vi "Latest File Check.vi"(5 "Target File Path":string, 7 "Initial File Path":string, 8 "error in (no error)":errorcluster, 9 "Matched Folder":string, 10 "Initial body in":string, 11 "Refnum in":T1) -> (0 "error out":errorcluster, 1 "body out":string, 2 "File Path Out":string, 3 "Refnum out":T1)   [LabVIEW 2019]
uses:
  <vilib>/httpClient/ClientHandle.ctl
  <vilib>/httpClient/LabVIEWHTTPClient.lvlib
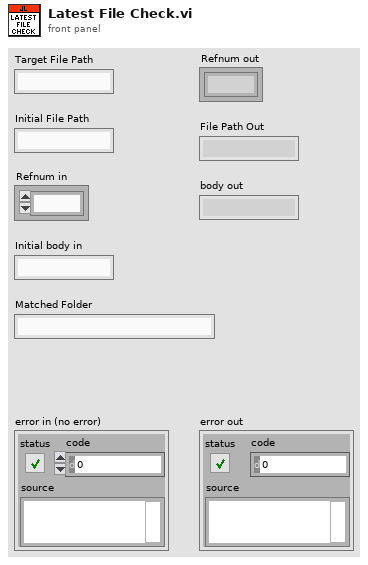
[diagram p1: front panel]
types:
  T1 = typedef "LabVIEWHTTPClient.lvlib/ClientHandle.ctl" = refnum<k1>
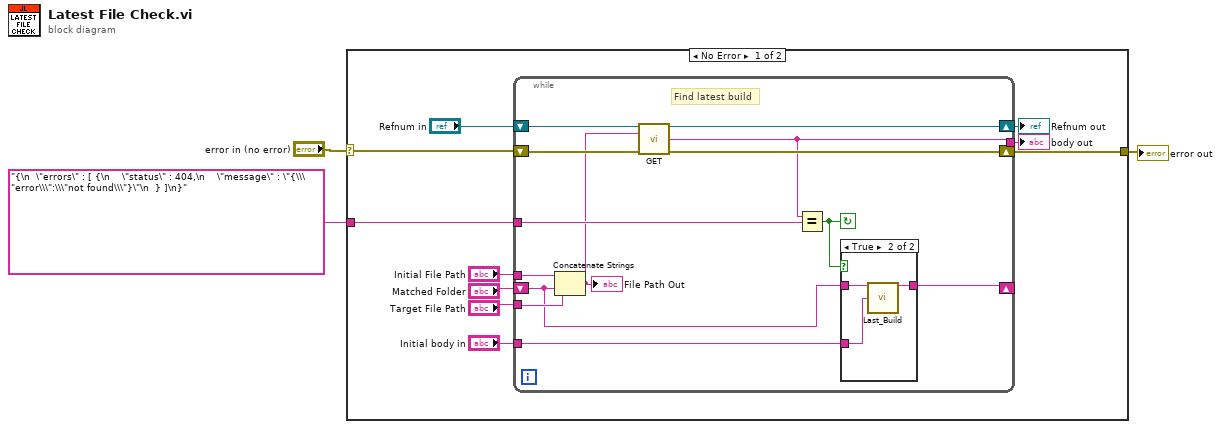
[diagram p0: block diagram]
diagram:
  n1 = case shown="No Error" "error in (no error)" {
    selector: "error in (no error)" -> [w6 w31]
    tunnel: "{\n  \"errors\" : [ {\n    \"status\" : 404,\n    \"message\" : \"{\\\"error\\\":\\\"not found\\\"}\"\n  } ]\n}" -> [w7 _]
    tunnel: [w4 w31] -> w1
    frame No Error {
      n2 = while {
        tunnel: "Initial File Path" -> [w26]
        shift-right: [w24] -> w4
        shift-left: w6 -> [w25]
        shift-right: [w21] -> w11
        shift-left: "Refnum in" -> [w22]
        tunnel: "Target File Path" -> [w23]
        shift-right: [w19] -> _
        shift-left: "Matched Folder" -> [w14]
        tunnel: "Initial body in" -> [w18]
        tunnel: w7 -> [w17]
        tunnel: [w15] -> w5
        stop <- w20 continue-if-true
        # "Find latest build"
        n3 = Concatenate Strings(w26, w14, w23) -> (w16:string)
        "File Path Out" <- w16
        n4 = call <vilib>:"GET.vi"("client handle"=w22, "url"=w16, "error in (no error)"=w25) -> ("client handle out"=w21:T1, "body"=w15:string, "error out"=w24:errorcluster)  [unwired: 9 in, 1 out]
        n5 = Equal?(x=w15, y=w17) -> (x = y?=w20:bool)
        n6 = case shown="True" w20 {
          tunnel: w18 -> [_ w30]
          tunnel: w14 -> [w27 w29]
          tunnel: [w27 w28] -> w19
          frame False {
          }
          frame True {
            n7 = call "Last_Build.vi"("Current Build"=w29, "Webpage Source"=w30) -> ("Next Build"=w28:string)  [unwired: 13 in]
          }
        }
      }
      "Refnum out" <- w11
      "body out" <- w5
    }
    frame Error {
    }
  }
  "error out" <- w1
